vi "Public Request.vi"(6 "timeout in ms":i32=-1, 8 "error in (no error)":errorcluster, 9 "Request Message Data":variant, 10 "Request Message":string, 11 "Mock Process In":refnum<class "Mock Process.lvclass">) -> (0 "error out":errorcluster, 1 "Response Message Data":variant, 2 "Response Message":string, 3 "Mock Process Out":refnum<class "Mock Process.lvclass">, 4 "Timed out?":bool)   [LabVIEW 2020, in "Mock Process.lvclass"]
uses:
  Mock Process.lvclass
  C:/Git/astemes-triarc-framework/source/Framework/Process/Process.lvclass
  Framework/Process/Process.lvclass/Process.ctl
  Framework/Process/Public/Lifecycle/Get Lifecycle State.vi
  Framework/Process/Private/SubVIs/Handle Debug Data.vi
  Framework/Process/Private/SubVIs/Enqueue Request Message.vi
  <vilib>/Utility/error.llb/Clear Errors.vi
  Framework/Logging/Log Debug.vi
  <vilib>/AdvancedString/1D String Array to Delimited String.vi
  <vilib>/Utility/High Resolution Relative Seconds.vi
  <vilib>/Utility/error.llb/Error Cluster From Error Code.vi
  Framework/Process/Public/Read Name.vi
  Framework/Process/Private/SubVIs/Wait for Response Message.vi
  Framework/Process/Process.lvclass
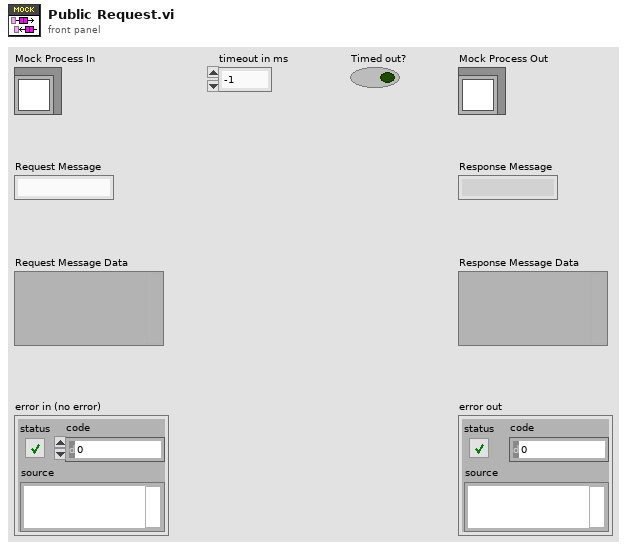
[diagram p1: front panel]
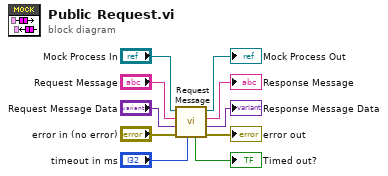
[diagram p0: block diagram]
diagram:
  n1 = call "Request Message.vi"("timeout in ms (-1)"="timeout in ms", "error in (no error)"="error in (no error)", "Request Message Data"="Request Message Data", "Request Message"="Request Message", "Process In"="Mock Process In") -> ("error out"=→"error out":errorcluster, "Response Message Data"=→"Response Message Data":variant, "Response Message"=→"Response Message":string, "Process Out"=→"Mock Process Out":refnum<class "Mock Process.lvclass">, "Timed out?"=→"Timed out?":bool)  [unwired: 2 in]
